vi "Read Channel Names.vi"(8 "error in":errorcluster, 10 "group name":string="Untitled", 11 "Data record":T1) -> (0 "error out":errorcluster, 3 "Data record out":T1)   [LabVIEW 2015]
uses:
  Controls/Data Viewer Entry.ctl
  Controls/Channel name entry.ctl
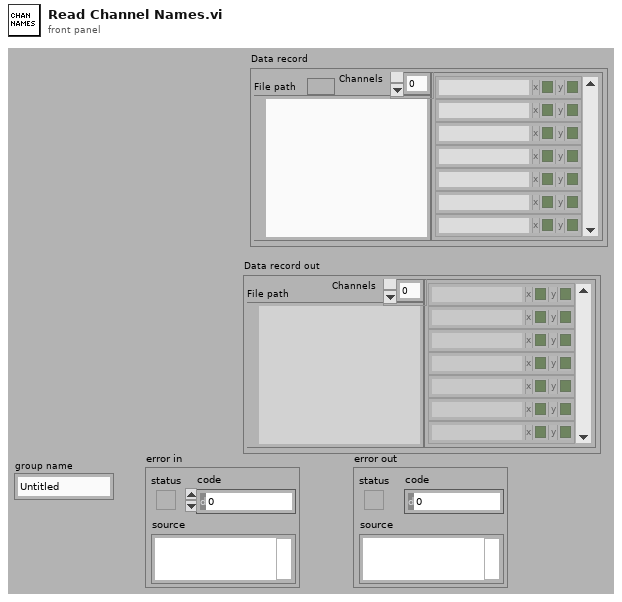
[diagram p1: front panel]
types:
  T1 = typedef "Data Viewer Entry.ctl" = cluster{"File path":path, "Channels":T2[]}
  T2 = typedef "Channel name entry.ctl" = cluster{"Name":string, "x":bool, "y":bool}
  T3 = enum16{"open", "open or create", "create or replace", "create", "open (read-only)"}
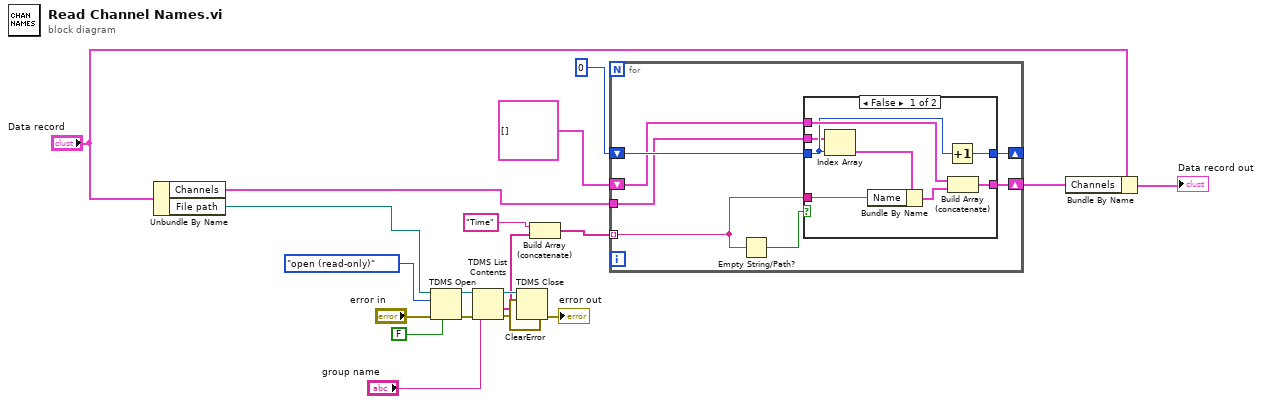
[diagram p0: block diagram]
diagram:
  n1 = Unbundle By Name("Data record") -> ("Channels"=w10:T2[], "File path"=w11:path)
  n2 = TDMS Open(6:FALSE ("disable buffering (T)"), 8:"error in", 10:T3."open (read-only)" ("operation (0:open)"), 11:w11) -> (0:w15:errorcluster, 3:w14:refnum<k34>)  [unwired: 3 in]
  n3 = TDMS List Contents(4:w15, 6:"group name", 7:w14) -> (0:w1:errorcluster, 1:w4:string[], 3:w13:refnum<k34>)  [unwired: 1 out]
  n4 = call <vilib>:"ClearError.vi"("error in (no error)"=w1) -> ("error out"=w12:errorcluster)
  n5 = TDMS Close(8:w12, 11:w13) -> (0:→"error out":errorcluster)  [unwired: 1 out]
  n6 = Build Array (concatenate)("Time", w4) -> (w3:string[])
  n7 = for {
    tunnel: w3 -> [w21] mode=indexing
    shift-right: [w25] -> _
    shift-left: 0 -> [w26]
    shift-right: [w24] -> w7
    shift-left: T2[] [] -> [w23]
    tunnel: w10 -> [w22]
    n8 = Empty String/Path?(string/path=w21) -> (empty?=w27:bool)
    n9 = case shown="False" w27 {
      tunnel: w21 -> [w35 _]
      tunnel: [w32 w36] -> w24
      tunnel: w26 -> [w30 w37]
      tunnel: [w34 w37] -> w25
      tunnel: w23 -> [w31 w36]
      tunnel: w22 -> [w29 _]
      frame False {
        n10 = Index Array(array=w29, index=w30) -> (element=w33:T2)
        n11 = Bundle By Name(cluster=w33, "Name"=w35) -> (w28:T2)
        n12 = Increment(x=w30) -> (x+1=w34:i32)
        n13 = Build Array (concatenate)(w31, w28) -> (w32:T2[])
      }
      frame True {
      }
    }
  }
  n14 = Bundle By Name(cluster="Data record", "Channels"=w7) -> (→"Data record out":T1)
